vi "IO_QueryCOM.vi"() -> ()   [LabVIEW 2024]
uses:
  <vilib>/Instr/_visa.llb/VISA Find Search Mode.ctl
  <vilib>/Utility/error.llb/Trim Whitespace One-Sided.vi
panel:
  out "Expected COM Port":refnum<visa-resource-name>
  out "Read Buffer":string
  out "Find List":string[](array[string])
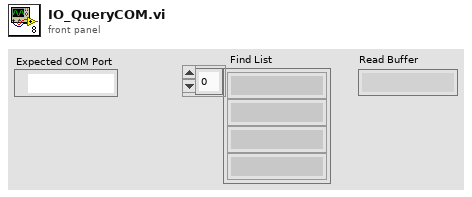
[diagram p1: front panel]
types:
  T1 = typedef "VISA Find Search Mode.ctl" = u32
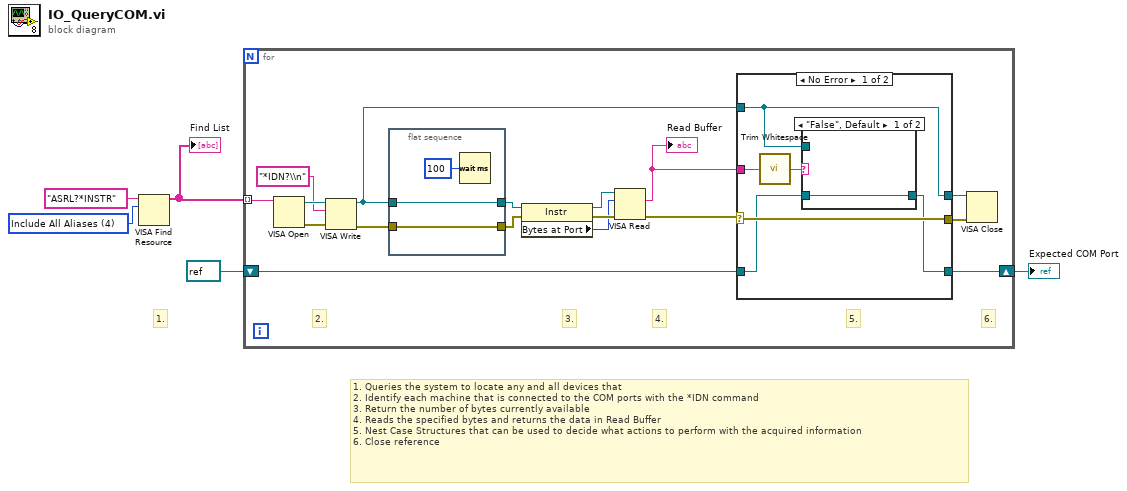
[diagram p0: block diagram]
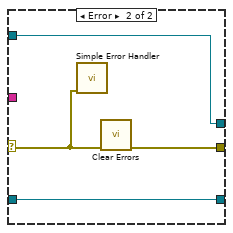
[diagram p3: hidden frame]
diagram:
  w2 = T1 4 items=["Canonical Names Only"=0, "Aliases Only"=2, "Include Matching Aliases"=3, "Include All Aliases"=4] ("Search Mode")
  # "1. Queries the system to locate any and all devices that \n2. Identify each machine that is connected to the COM ports with the *IDN command\n3. Return the number of bytes currently available\n4. Reads the specified bytes and returns the data in Read Buffer\n5. Nest Case Structures that can be used to decide what actions to perform with the acquired information\n6. Close reference"
  # "1."
  n1 = VISA Find Resource(10:w2, 11:"ASRL?*INSTR" ("expression (\"?*\")")) -> (3:w1:string[])  [unwired: 1 in, 2 out]
  "Find List" <- w1
  n2 = for {
    tunnel: w1 -> [w22] mode=indexing
    shift-right: [w6] -> w3
    shift-left: refnum<visa-resource-name> refnum ("VISA resource name out") -> [w7]
    # "6."
    # "5."
    # "4."
    # "3."
    # "2."
    n3 = VISA Open(VISA resource name=w22) -> (VISA resource name=w21:refnum<visa-resource-name>, error out=w20:errorcluster)  [unwired: 4 in]
    n4 = VISA Write(VISA resource name=w21, write buffer="*IDN?\\n", error in (no error)=w20) -> (VISA resource name out=w11:refnum<visa-resource-name>, error out=w19:errorcluster)  [unwired: 1 out]
    n5 = flat-sequence {
      tunnel: w11 -> [w24]
      tunnel: [w24] -> w17
      tunnel: w19 -> [w23]
      tunnel: [w23] -> w16
      frame #0 {
        n6 = Wait (ms)(milliseconds to wait=u32 100) -> ()  [unwired: 1 out]
      }
    }
    n7 = property class="Instr"(reference=w17, error in=w16) -> (reference out=w8:refnum<visa-resource-name>, error out=w15:errorcluster, "Bytes at Port"=w9:u32)
    n8 = VISA Read(VISA resource name=w8, byte count=w9, error in (no error)=w15) -> (read buffer=w10:string, error out=w14:errorcluster)  [unwired: 2 out]
    "Read Buffer" <- w10
    n9 = case shown="No Error" w14 {
      selector: w14 -> [w31 w34]
      tunnel: [w31 w36] -> w13
      tunnel: [w28 w37] -> w12
      tunnel: w11 -> [w28 w37]
      tunnel: w10 -> [w30 _]
      tunnel: w7 -> [w27 w35]
      tunnel: [w26 w35] -> w6
      frame No Error {
        n10 = call <vilib>:"Trim Whitespace.vi"("string"=w30) -> ("trimmed string"=w29:string)  [unwired: 1 in]
        n11 = case shown="\"False\", Default" w29 {
          tunnel: w28 -> [_ w33]
          tunnel: [w32 w33] -> w26
          tunnel: w27 -> [w32 _]
          frame "False", Default {
          }
          frame "00062" {
          }
        }
      }
      frame Error {
        n12 = call <vilib>:"Simple Error Handler.vi"("error in (no error)"=w34) -> ()  [unwired: 4 in, 5 out]
        n13 = call <vilib>:"Clear Errors.vi"("error in (no error)"=w34) -> ("error out"=w36:errorcluster)  [unwired: 5 in, 1 out]
      }
    }
    n14 = VISA Close(VISA resource name=w12, error in (no error)=w13) -> ()  [unwired: 1 out]
  }
  "Expected COM Port" <- w3
